vi "getFastMessages.vi"(8 "error in (no error)":errorcluster, 11 "AlCS in":refnum<class "AlCS.lvclass">) -> (0 "error out":errorcluster, 2 "message":string, 3 "AlCS out":refnum<class "AlCS.lvclass">)   [LabVIEW 2016, in "AlCS.lvclass"]
uses:
  AlCS.lvclass
  AlCS.lvclass/AlCS.ctl
  ts_labview_tcp/TCPClient/TCPClient.lvclass
  ts_labview_tcp/TCPSettings/TCPSettings.lvclass
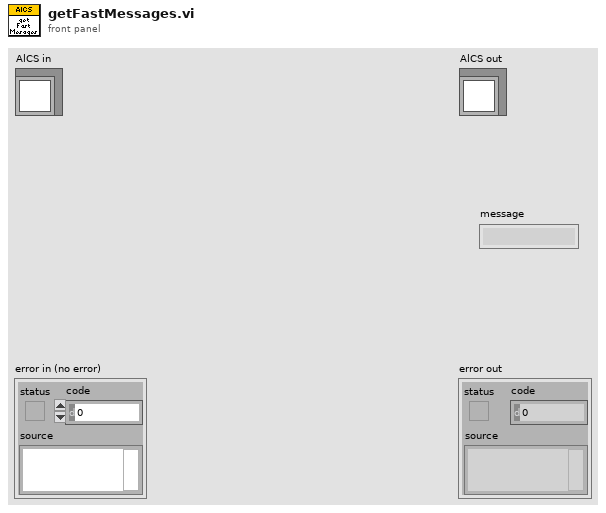
[diagram p1: front panel]
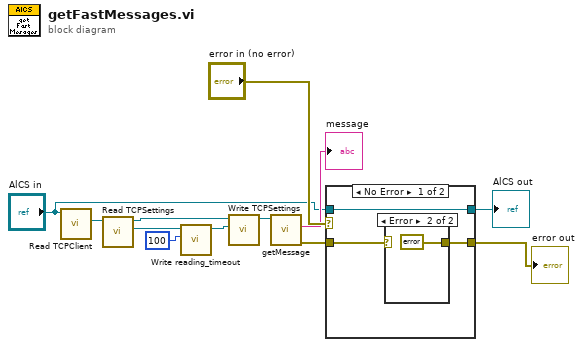
[diagram p0: block diagram]
diagram:
  n1 = call "Read TCPClient.vi"("AlCS in"="AlCS in") -> ("TCPClient.lvclass"=w7:refnum<class "TCPClient.lvclass">)  [unwired: 8 in, 2 out]
  n2 = call-dynamic "Read TCPSettings.vi"("TCPCommunicator in"=w7) -> ("TCPSettings.lvclass"=w6:refnum<class "TCPSettings.lvclass">, "TCPCommunicator out"=w3:refnum<class "TCPClient.lvclass">)  [unwired: 8 in, 1 out]
  n3 = call-dynamic "Write reading_timeout.vi"("reading_timeout"=100, "TCPSettings in"=w6) -> ("TCPSettings out"=w4:refnum<class "TCPSettings.lvclass">)  [unwired: 8 in, 1 out]
  n4 = call-dynamic "Write TCPSettings.vi"("TCPSettings.lvclass"=w4, "TCPCommunicator in"=w3) -> ("TCPCommunicator out"=w2:refnum<class "TCPClient.lvclass">)  [unwired: 8 in, 1 out]
  n5 = call-dynamic "getMessage.vi"("TCPClient in"=w2) -> ("error out"=w12:errorcluster, "String"=→"message":string)  [unwired: 8 in, 1 out]
  n6 = case shown="No Error" "error in (no error)" {
    selector: "error in (no error)" -> [_ w19]
    tunnel: [w13 w19] -> w1
    tunnel: [w15 w18] -> w8
    tunnel: "AlCS in" -> [w15 w18]
    tunnel: w12 -> [w14 _]
    frame No Error {
      n7 = case shown="Error" w14 {
        selector: w14 -> [w16 _]
        tunnel: [w16 errorcluster {"status"=TRUE, "code"=8204, "source"="Monochromator Controller not responding"} ("error IO")] -> w13
        frame No Error {
        }
        frame Error {
        }
      }
    }
    frame Error {
    }
  }
  "error out" <- w1
  "AlCS out" <- w8
